vi "Get Picture Ring Solution.vi"(8 "error in (no error)":errorcluster, 11 "Grassfire 2D In":refnum<class "Grassfire 2D.lvclass">) -> (0 "error out":errorcluster, 2 "Array":T1[][](array[typedef]), 3 "Grassfire 2D Out":refnum<class "Grassfire 2D.lvclass">)   [LabVIEW 2019, in "Grassfire 2D.lvclass"]
uses:
  Grassfire 2D.lvclass
  Shared/Solution Node--cluster.ctl
  Shared/Solution--picture ring.ctl
  Grassfire 2D.lvclass/Grassfire 2D.ctl
  Shared/Shared.lvlib
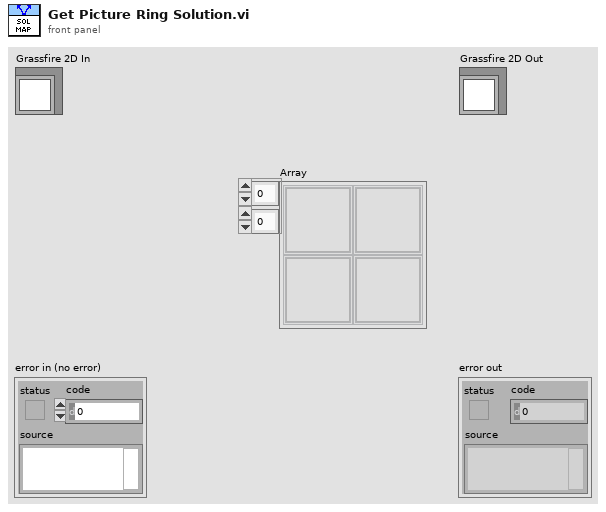
[diagram p1: front panel]
types:
  T1 = typedef "Shared.lvlib/Solution Node--cluster.ctl" = cluster{"Type":T2, "Distance":string}
  T2 = typedef "Shared.lvlib/Solution--picture ring.ctl" = i64
  T3 = typedef "Grassfire 2D.lvclass/Node Address--cluster.ctl" = cluster{"Row":i32, "Column":i32}
  T4 = typedef "Grassfire 2D.lvclass/Node Value--cluster.ctl" = cluster{"Type":T5, "Distance":i32}
  T5 = typedef "Shared.lvlib/Node Type--enum.ctl" = enum16{"Empty", "Blocked", "Start", "End", "Path"}
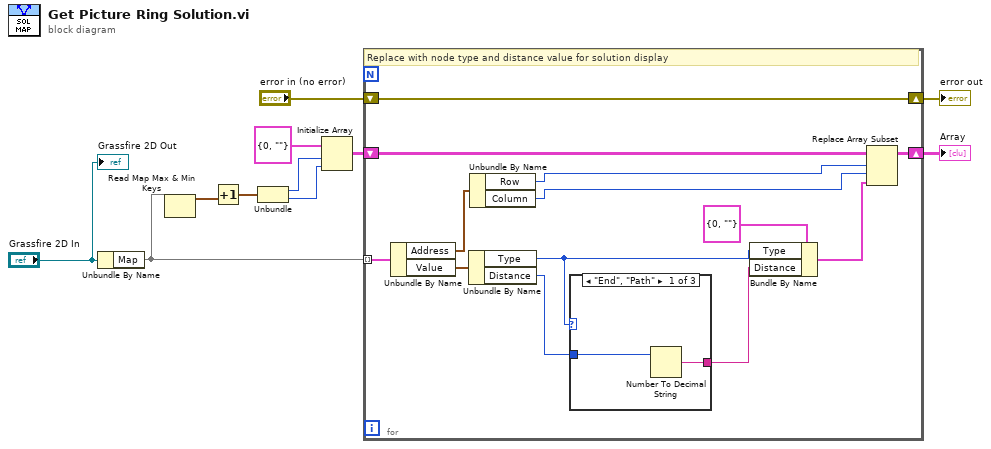
[diagram p0: block diagram]
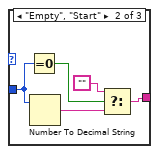
[diagram p2: hidden frame]
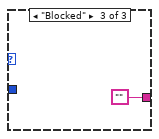
[diagram p3: hidden frame]
diagram:
  n1 = Unbundle By Name("Grassfire 2D In") -> ("Map"=w10:map{T3, T4})
  n2 = Read Map Max & Min Keys(11:w10) -> (3:w5:T3)  [unwired: 1 out]
  n3 = Increment(x=w5) -> (x+1=w4:T3)
  n4 = Unbundle(w4) -> ("Row"=w3:i32, "Column"=w2:i32)
  n5 = Initialize Array(T1 {"Type"=0, "Distance"=""} ("Cell"), w3, w2) -> (w11:T1[][])
  n6 = for {
    shift-right: [w23] -> w6
    shift-left: w11 -> [w24]
    tunnel: w10 -> [w18] mode=indexing
    shift-right: [w22] -> w7
    shift-left: "error in (no error)" -> [w22]
    # "Replace with node type and distance value for solution display"
    n7 = Unbundle By Name(w18) -> ("Address"=w14:T3, "Value"=w17:T4)
    n8 = Unbundle By Name(w17) -> ("Type"=w16:T5, "Distance"=w15:i32)
    n9 = Unbundle By Name(w14) -> ("Row"=w13:i32, "Column"=w12:i32)
    n10 = case shown="\"End\", \"Path\"" w16 {
      tunnel: w15 -> [w26 w31 _]
      tunnel: [w25 w27 ""] -> w20
      frame "End", "Path" {
        n11 = Number To Decimal String(number=w26) -> (decimal integer string=w25:string)  [unwired: 1 in]
      }
      frame "Empty", "Start" {
        n12 = Equal To 0?(x=w31) -> (x = 0?=w30:bool)
        n13 = Number To Decimal String(number=w31) -> (decimal integer string=w28:string)  [unwired: 1 in]
        n14 = Select(t="", s=w30, f=w28) -> (s? t:f=w27:string)
      }
      frame "Blocked" {
      }
    }
    n15 = Bundle By Name(cluster=T1 {"Type"=0, "Distance"=""} ("Cell"), "Type"=w16, "Distance"=w20) -> (w21:T1)
    n16 = Replace Array Subset(array=w24, new element=w21, index (row)=w13, index (col)=w12) -> (w23:T1[][])
  }
  "error out" <- w7
  "Array" <- w6
  "Grassfire 2D Out" <- "Grassfire 2D In"
